vi "Finish.vi"   [LabVIEW 2015]
doc: "This VI is called just before exiting. It is expected to close I/O refnum, save collected data, etc."
uses:
  <vilib>/Rock Robotics/WPI/Utilities/WPI_GetSetVariantRefNum.vi
types:
  T1 = typedef "WPI_JoystickDevRef.ctl" = cluster{"Device":T2}
  T2 = typedef "WPI_JoystickDeviceEnum.ctl" = enum16{"USB 0", "USB 1", "USB 2", "USB 3", "USB 4", "USB 5"}
  T3 = typedef "Motor_Type_Def.ctl" = cluster{"Drive_Motor":cluster{"RobotDriveDevRef":T4, "error out":errorcluster}, "Intake_1":cluster{"MotorControlDevRef":T5, "error out":errorcluster}, "Intake_Stage":cluster{"MotorControlDevRef":T5, "error out":errorcluster}, "Shooter_Motor_1":cluster{"MotorControlDevRef":T5, "error out":errorcluster}}
  T4 = typedef "WPI_RobotDriveDevRef.ctl" = cluster{"DevStatus":errorcluster, "Motors[]":T5[], "Square Inputs":bool, "Max Output":dbl}
  T5 = typedef "WPI_MotorControlDeviceRef.ctl" = cluster{"DeviceStatus":errorcluster, "Type":T6, "PWM":cluster{"PWM Channel":T7, "DeadBand":T8}, "CAN":cluster{"Device Number":u8, "Control Mode":T9, "Semaphore":T10, "Max Vout":dbl, "TalonSRX Control Mode":T11}, "Invert":bool}
  T6 = typedef "WPI_MotorControlType.ctl" = enum16{"PWM", "CAN", "CANTalonSRX"}
  T7 = typedef "FPGA_DIOPWMChannel.ctl" = enum8{"PWM 0", "PWM 1", "PWM 2", "PWM 3", "PWM 4", "PWM 5", "PWM 6", "PWM 7", "PWM 8", "PWM 9", "PWM MXP 0", "PWM MXP 1", "PWM MXP 2", "PWM MXP 3", "PWM MXP 4", "PWM MXP 5", "PWM MXP 6", "PWM MXP 7", "PWM MXP 8", "PWM MXP 9", "Invalid"}
  T8 = typedef "WPI_PWMDeadband.ctl" = cluster{"Name":string, "maxPositivePwm":i32, "minPositivePwm":i32, "centerPwm":i32, "maxNegativePwm":i32, "minNegativePwm":i32, "angularRange":u16}
  T9 = typedef "WPI_CANJaguar_ControlMode.ctl" = enum8{"Percent VBus", "Current", "Speed", "Position", "Voltage"}
  T10 = typedef "Semaphore RefNum" = refnum<k1>
  T11 = typedef "WPI_CANTalonSRX_APIControlMode.ctl" = enum8{"Percent VBus", "Speed", "Position", "Slave", "Unchanged / Invalid", "Voltage Compensation", "Current", "Motion Profile"}
  T12 = typedef "Pneu_Type_Def.ctl" = cluster{"Intake_Arm":cluster{"SolenoidDevRef":T13, "error out":errorcluster}, "Gear":cluster{"SolenoidDevRef":T13, "error out":errorcluster}, "Flipper":cluster{"SolenoidDevRef":T13, "error out":errorcluster}, "Arm_defense":cluster{"SolenoidDevRef":T13, "error out":errorcluster}, "Compressor":cluster{"CompressorDevRef":T15, "error out":errorcluster}}
  T13 = typedef "WPI_SolenoidDevRef.ctl" = cluster{"DevStatus":errorcluster, "Pneumatics Control Module":u8, "Forward Solenoid Channel":T14, "Reverse Solenoid Channel":T14}
  T14 = typedef "WPI_SolenoidChannel.ctl" = enum8{"Solenoid 0", "Solenoid 1", "Solenoid 2", "Solenoid 3", "Solenoid 4", "Solenoid 5", "Solenoid 6", "Solenoid 7", "Invalid"}
  T15 = typedef "WPI_CompressorDevRef.ctl" = cluster{"DevStatus":errorcluster, "Pneumatics Control Module":u8}
  T16 = typedef "DIO_Type_Def.ctl" = cluster{"Left_Back":cluster{"SonarMB1010DigitalDevRef":T17, "error out":errorcluster}, "Left_Front":cluster{"SonarMB1010DigitalDevRef":T17, "error out":errorcluster}, "Right_Back":cluster{"SonarMB1010DigitalDevRef":T17, "error out":errorcluster}, "Right_Front":cluster{"SonarMB1010DigitalDevRef":T17, "error out":errorcluster}, "Front":cluster{"SonarMB1010DigitalDevRef":T17, "error out":errorcluster}, "Left Encoder":cluster{"EncoderDevRef":T20, "error out":errorcluster}, "Right Encoder":cluster{"EncoderDevRef":T20, "error out":errorcluster}, "Shooter Encoder":cluster{"CounterDevRef":T18, "error out":errorcluster}, "Intake_Storing":cluster{"DigitalInputDevRef":T23, "error out":errorcluster}, "Intake_Staged":cluster{"DigitalInputDevRef":T23, "error out":errorcluster}}
  T17 = typedef "WPI_SonarMB1010DigitalDeviceRef.ctl" = cluster{"CounterDevRef":T18, "Scaling factor (s/in)":dbl}
  T18 = typedef "WPI_CounterDevRef.ctl" = cluster{"DevStatus":errorcluster, "CntIndex":T19}
  T19 = typedef "FPGA_CounterCtrSystemIndex.ctl" = enum8{"Ctr 0", "Ctr 1", "Ctr 2", "Ctr 3", "Ctr 4", "Ctr 5", "Ctr 6", "Ctr 7", "Invalid"}
  T20 = typedef "WPI_EncoderDevRef.ctl" = cluster{"DevStatus":errorcluster, "EncoderIndex":T21, "CounterIndex":T19, "DistancePerCount":dbl, "Decoding Type":T22}
  T21 = typedef "FPGA_EncoderIdx.ctl" = enum8{"Enc 0", "Enc 1", "Enc 2", "Enc 3", "Enc 4", "Enc 5", "Enc 6", "Enc 7", "Invalid"}
  T22 = typedef "WPI_EncoderType.ctl" = enum16{"1x", "2x", "4x"}
  T23 = typedef "WPI_DigitalInputDevRef.ctl" = cluster{"DevStatus":errorcluster, "DIO Channel":T24}
  T24 = typedef "FPGA_DIOChannel.ctl" = enum8{"DIO 0", "DIO 1", "DIO 2", "DIO 3", "DIO 4", "DIO 5", "DIO 6", "DIO 7", "DIO 8", "DIO 9", "DIO MXP 0", "DIO MXP 1", "DIO MXP 2", "DIO MXP 3", "DIO MXP 4", "DIO MXP 5", "DIO MXP 6", "DIO MXP 7", "DIO MXP 8", "DIO MXP 9", "DIO MXP 10", "DIO MXP 11", "DIO MXP 12", "DIO MXP 13", "DIO MXP 14", "DIO MXP 15", "Invalid"}
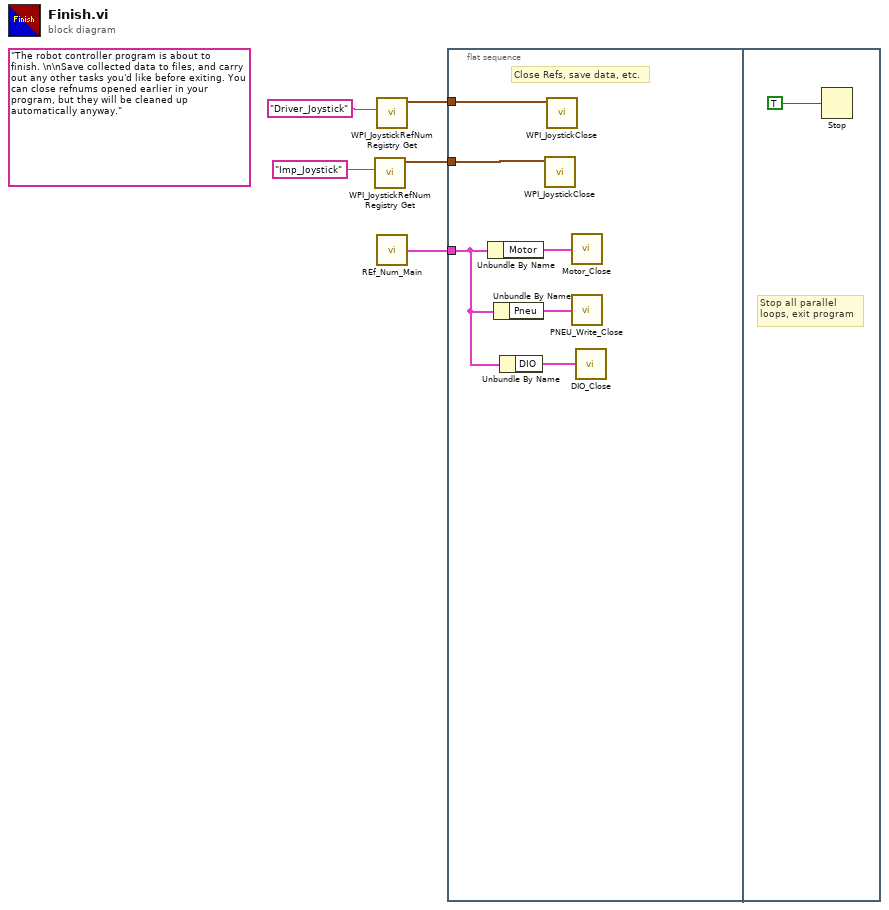
[diagram p0: block diagram]
diagram:
  (unwired) "The robot controller program is about to finish. \n\nSave collected data to files, and carry out any other tasks you'd like before exiting. You can close refnums opened earlier in your program, but they will be cleaned up automatically anyway."
  n1 = call <vilib>:"WPI_JoystickRefNum Registry Get.vi"("refnum name"="Imp_Joystick") -> ("JoystickDevRef"=w3:T1)  [unwired: 1 in, 9 out]
  n2 = call <vilib>:"WPI_JoystickRefNum Registry Get.vi"("refnum name"="Driver_Joystick") -> ("JoystickDevRef"=w5:T1)  [unwired: 1 in, 9 out]
  n3 = call "REf_Num_Main.vi"() -> ("Ref_Num"=w4:cluster{"Motor":T3, "Pneu":T12, "DIO":T16})
  n4 = flat-sequence {
    tunnel: w5 -> [w11]
    tunnel: w4 -> [w7]
    tunnel: w3 -> [w8]
    frame #0 {
      # "Close Refs, save data, etc."
      n5 = Unbundle By Name(w7) -> ("Motor"=w10:T3)
      n6 = Unbundle By Name(w7) -> ("Pneu"=w9:T12)
      n7 = Unbundle By Name(w7) -> ("DIO"=w6:T16)
      n8 = call <vilib>:"WPI_JoystickClose.vi"("JoystickDevRef"=w8) -> ()  [unwired: 11 out]
      n9 = call <vilib>:"WPI_JoystickClose.vi"("JoystickDevRef"=w11) -> ()  [unwired: 11 out]
      n10 = call "Motor_Close.vi"("Motor"=w10) -> ()
      n11 = call "PNEU_Write_Close.vi"("Pneu"=w9) -> ()
      n12 = call "DIO_Close.vi"("output cluster 3"=w6) -> ()
    }
    frame #1 {
      # "Stop all parallel\nloops, exit program"
      n13 = Stop(stop? (T)=TRUE ("Quit")) -> ()
    }
  }
